vi "Rename Caption.vi"(8 "error in (no error)":errorcluster, 10 "Caption":string, 11 "GObject in":refnum<vi>) -> (0 "error out":errorcluster, 2 "has caption?":bool, 3 "GObject out":refnum<vi>)   [LabVIEW 2019, in "Builtins.lvlib"]
doc: "Renames the GObject caption if exists and moves the label to the appropriate position. If the caption is empty this does nothing. This hides the label if visible.\n\nCreated by: Ryan Pacini"
uses:
  Builtins.lvlib
  Label Position.ctl
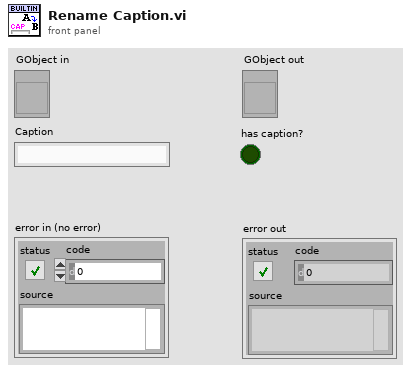
[diagram p1: front panel]
types:
  T1 = typedef "Builtins.lvlib/Label Position.ctl" = enum8{"Unchanged", "Top-left", "Top-middle", "Top-right", "Right-top", "Right-middle", "Right-bottom", "Bottom-right", "Bottom-middle", "Bottom-left", "Left-bottom", "Left-middle", "Left-top"}
  T2 = typedef "LVRectTypeDef.ctl" = cluster{"Left":i16, "Top":i16, "Right":i16, "Bottom":i16}
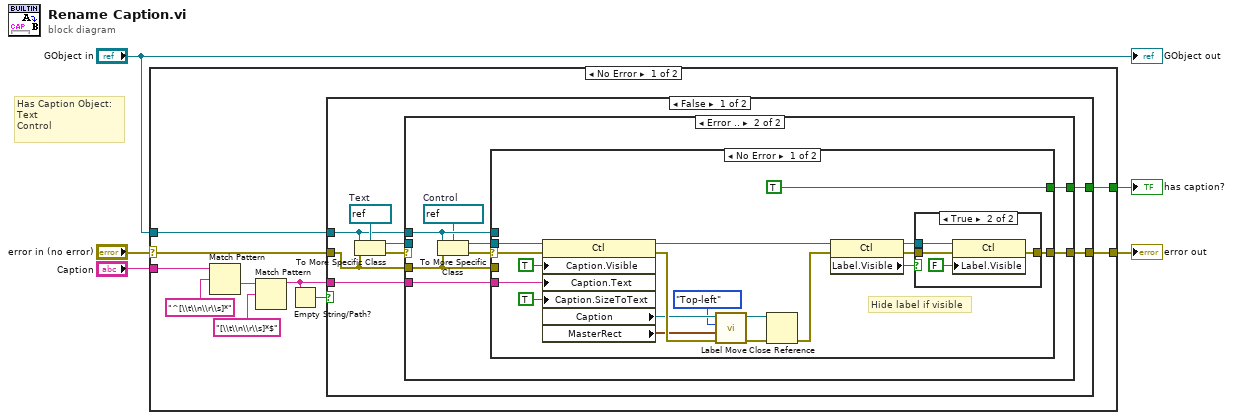
[diagram p0: block diagram]
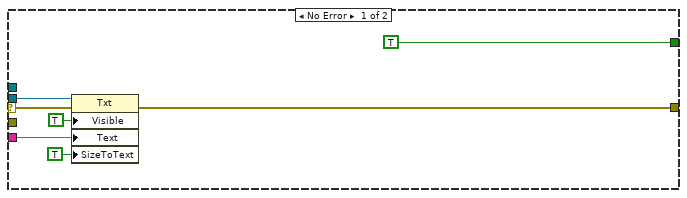
[diagram p2: hidden frame]
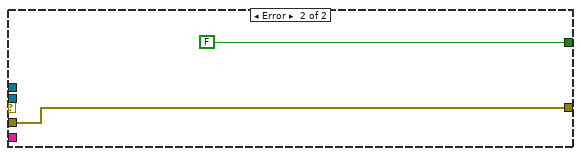
[diagram p4: hidden frame]
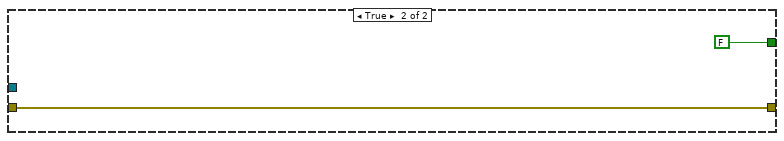
[diagram p5: hidden frame]
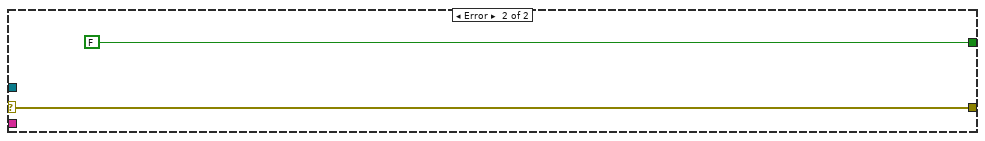
[diagram p6: hidden frame]
diagram:
  # "Has Caption Object:\nText\nControl"
  n1 = case shown="No Error" "error in (no error)" {
    selector: "error in (no error)" -> [w13 w67]
    tunnel: "GObject in" -> [w12 _]
    tunnel: [w15 w67] -> w1
    tunnel: [w14 FALSE] -> w2
    tunnel: "Caption" -> [w6 _]
    frame No Error {
      n2 = Match Pattern(string=w6, regular expression="^[\\t\\n\\r\\s]*") -> (after substring=w10:string)  [unwired: 1 in, 3 out]
      n3 = Match Pattern(string=w10, regular expression="[\\t\\n\\r\\s]*$") -> (before substring=w7:string)  [unwired: 1 in, 3 out]
      n4 = Empty String/Path?(string/path=w7) -> (empty?=w11:bool)
      n5 = case shown="False" w11 {
        tunnel: [w23 w65] -> w15
        tunnel: [w22 FALSE] -> w14
        tunnel: w7 -> [w21 _]
        tunnel: w13 -> [w19 w65]
        tunnel: w12 -> [w18 _]
        frame False {
          w20 = refnum<vi> refnum  # Text
          n6 = To More Specific Class(target class=w20, reference=w18, error in=w19) -> (specific class reference=w16:refnum<vi>, error out=w17:errorcluster)
          n7 = case shown="Error .." w17 {
            selector: w17 -> [w29 _]
            tunnel: [w26 w38] -> w23
            tunnel: [TRUE w37] -> w22
            tunnel: w19 -> [_ w36]
            tunnel: w18 -> [_ w35]
            tunnel: w21 -> [w28 w34]
            tunnel: w16 -> [w30 _]
            frame No Error {
              n8 = property class="Txt"(reference=w30, error in=w29, "Visible"=TRUE, "Text"=w28, "SizeToText"=TRUE ("Size to Text?")) -> (error out=w26:errorcluster)  [unwired: 1 out]
            }
            frame Error {
              w31 = refnum<vi> refnum  # Control
              n9 = To More Specific Class(target class=w31, reference=w35, error in=w36) -> (specific class reference=w32:refnum<vi>, error out=w33:errorcluster)
              n10 = case shown="No Error" w33 {
                selector: w33 -> [w56 _]
                tunnel: w32 -> [w55 _]
                tunnel: w35 -> [_ _]
                tunnel: w36 -> [_ w63]
                tunnel: [w42 w63] -> w38
                tunnel: [TRUE FALSE] -> w37
                tunnel: w34 -> [w54 _]
                frame No Error {
                  # "Hide label if visible"
                  n11 = property class="Ctl"(reference=w55, error in=w56, "Caption.Visible"=TRUE ("Label.Visible"), "Caption.Text"=w54, "Caption.SizeToText"=TRUE ("Caption.Size to Text?")) -> (reference out=w43:refnum<vi>, error out=w50:errorcluster, "Caption"=w48:refnum<vi>, "MasterRect"=w47:T2)
                  n12 = call "Label Move.vi"("error in (no error)"=w50, "Owner Master Bounds Rect"=w47, "Label Position"=Label_Position."Top-left", "Label in"=w48) -> ("error out"=w52:errorcluster, "dup Label"=w51:refnum<vi>)  [unwired: 6 in]
                  n13 = Close Reference(reference=w51, error in (no error)=w52) -> (error out=w49:errorcluster)
                  n14 = property class="Ctl"(reference=w43, error in=w49) -> (reference out=w41:refnum<vi>, error out=w44:errorcluster, "Label.Visible"=w40:bool)
                  n15 = case shown="True" w40 {
                    tunnel: w44 -> [w57 w61]
                    tunnel: [w57 w60] -> w42
                    tunnel: w41 -> [_ w59]
                    frame False {
                    }
                    frame True {
                      n16 = property class="Ctl"(reference=w59, error in=w61, "Label.Visible"=FALSE) -> (error out=w60:errorcluster)  [unwired: 1 out]
                    }
                  }
                }
                frame Error {
                }
              }
            }
          }
        }
        frame True {
        }
      }
    }
    frame Error {
    }
  }
  "error out" <- w1
  "has caption?" <- w2
  "GObject out" <- "GObject in"
